vi "subWriteToFile.vi"(9 "Export string":string, 10 "Filename":string, 11 "Path":string) -> (0 "error out":errorcluster)   [LabVIEW 2020, in "DefaultExtensions.lvlib" / "CGrapherDGML.lvclass"]
uses:
  CGrapherDGML.lvclass
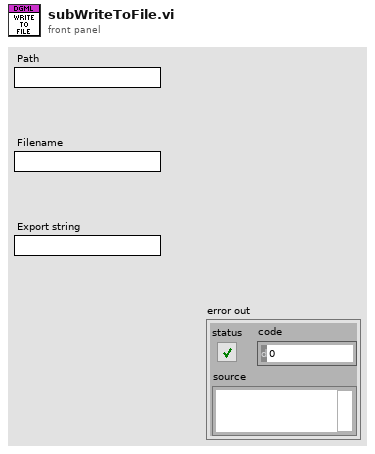
[diagram p1: front panel]
types:
  T1 = enum16{"open", "replace", "create", "open or create", "replace or create", "replace or create with confirmation"}
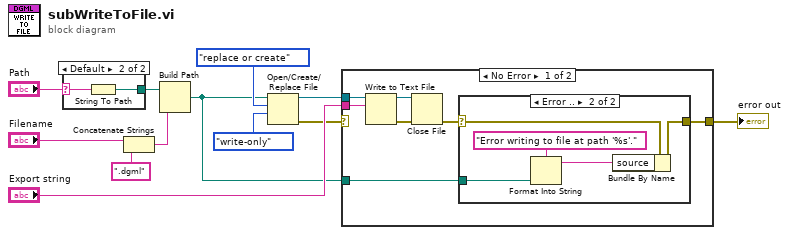
[diagram p0: block diagram]
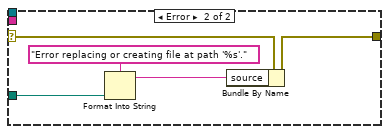
[diagram p3: hidden frame]
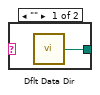
[diagram p4: hidden frame]
diagram:
  n1 = case shown="Default" "Path" {
    selector: "Path" -> [_ w14]
    tunnel: [w13 w15] -> w9
    frame "" {
      n2 = call <vilib>:"Dflt Data Dir.vi"() -> ("App:Default Data Directory"=w13:path)
    }
    frame Default {
      n3 = String To Path(string=w14) -> (path=w15:path)
    }
  }
  n4 = Concatenate Strings("Filename", ".dgml" ("string")) -> (w10:string)
  n5 = Build Path(base path=w9, name or relative path=w10) -> (appended path=w2:path)
  n6 = Open/Create/Replace File(file path (use dialog)=w2, operation (0:open)=T1."replace or create", access (0:read/write)=enum16{"read/write", "read-only", "write-only"}."write-only") -> (refnum out=w5:refnum<file>, error out=w6:errorcluster)  [unwired: 3 in, 1 out]
  n7 = case shown="No Error" w6 {
    selector: w6 -> [_ w33]
    tunnel: w5 -> [w22 _]
    tunnel: "Export string" -> [w20 _]
    tunnel: [w17 w32] -> w7
    tunnel: w2 -> [w16 w31]
    frame No Error {
      n8 = Write to Text File(file (use dialog)=w22, text=w20) -> (refnum out=w21:refnum<file>, error out=w19:errorcluster)  [unwired: 2 in, 1 out]
      n9 = Close File(refnum=w21, error in=w19) -> (error out=w18:errorcluster)  [unwired: 1 out]
      n10 = case shown="Error .." w18 {
        selector: w18 -> [w23 w26]
        tunnel: [w23 w25] -> w17
        tunnel: w16 -> [_ w24]
        frame No Error {
        }
        frame Error {
          n11 = Format Into String(format string="Error writing to file at path '%s'.", w24) -> (resulting string=w28:string)  [unwired: 2 in, 1 out]
          n12 = Bundle By Name(cluster=w26, "source"=w28) -> (w25:errorcluster)
        }
      }
    }
    frame Error {
      n13 = Format Into String(format string="Error replacing or creating file at path '%s'.", w31) -> (resulting string=w30:string)  [unwired: 2 in, 1 out]
      n14 = Bundle By Name(cluster=w33, "source"=w30) -> (w32:errorcluster)
    }
  }
  "error out" <- w7
